vi "MultipleResultsPanelModel-GFV.vi"(8 "error in (no error)":errorcluster, 10 "Data in":variant, 11 "Enum":T1=enum."Init") -> (0 "error out":errorcluster, 3 "Data out":variant)   [LabVIEW 2013]
doc: "Use this template to build a VI to use as a subVI."
uses:
  TypeDef/MultipleResultsDataModel.ctl
  TypeDef/MultipleResultsModelOutput.ctl
  TypeDef/MultipleFilesModelInput.ctl
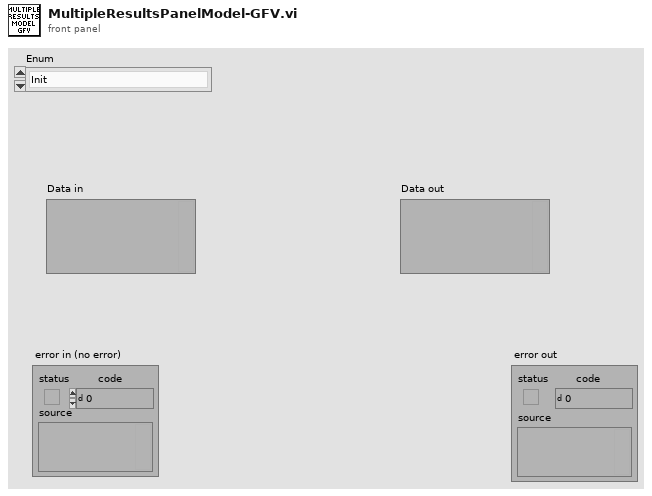
[diagram p1: front panel]
types:
  T1 = typedef "MultipleResultsDataModel.ctl" = enum16{"Get Results DB", "Get Plot Names", "Add Result File", "Init", "Get Input Data", "Get Result Graph Data", "Save Results DB", "Save Input Data"}
  T2 = typedef "MultipleResultsModelOutput.ctl" = cluster{"Ramp Pattern":dbl[], dbl[], "Include graph":bool, "Graph Name":string}[]
  T3 = typedef "MultipleFilesModelInput.ctl" = cluster{"Min Diameter (µm)":dbl, "Max Diameter (µm)":dbl, "FilterDropletsFrozeBelow":dbl, "Temperature offset for Calibration":dbl, "BinSizeDeg":dbl}
  T4 = cluster{"Values":dbl[][], "filename without extension":string}
  T5 = cluster{"Ramp Pattern":dbl[], dbl[], "Include graph":bool, "Graph Name":string}
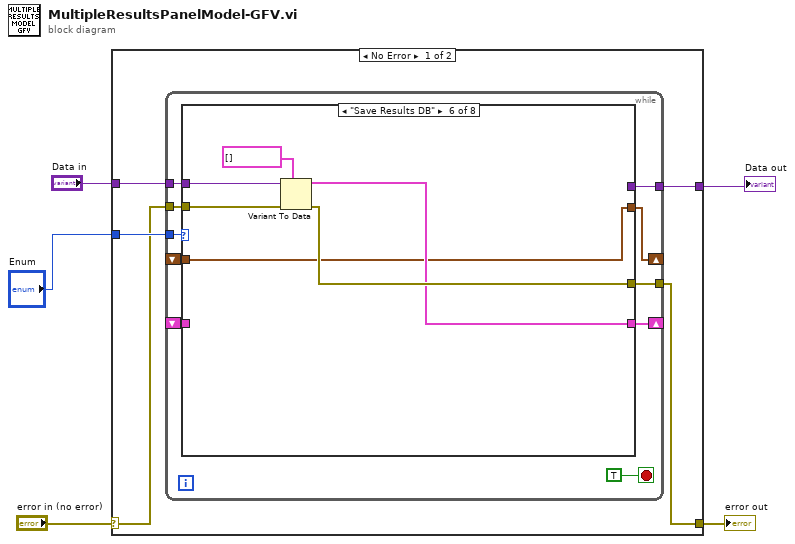
[diagram p0: block diagram]
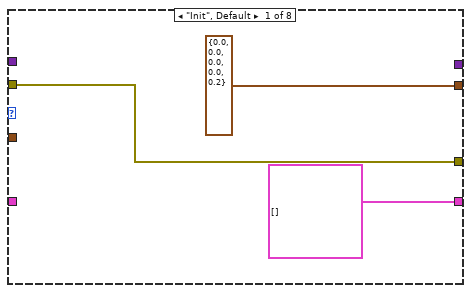
[diagram p2: hidden frame]
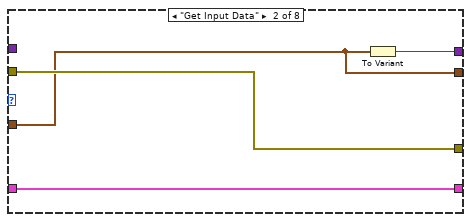
[diagram p3: hidden frame]
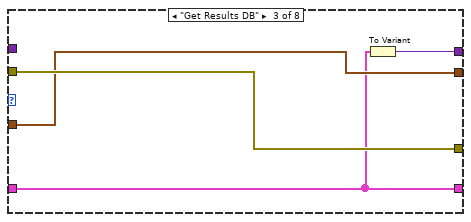
[diagram p4: hidden frame]
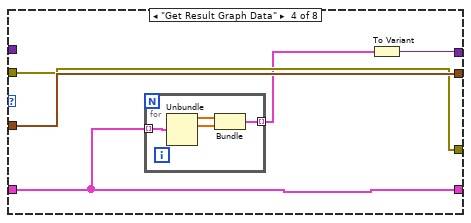
[diagram p5: hidden frame]
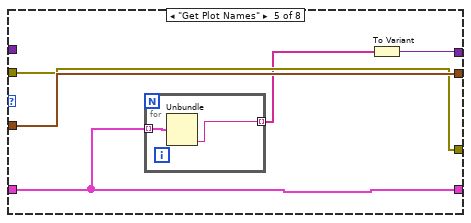
[diagram p6: hidden frame]
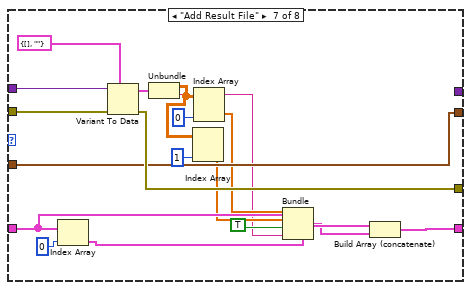
[diagram p7: hidden frame]
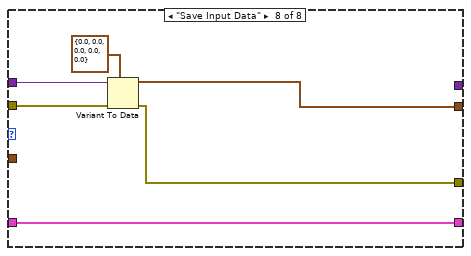
[diagram p8: hidden frame]
diagram:
  n1 = case shown="No Error" "error in (no error)" {
    selector: "error in (no error)" -> [w8 w78]
    tunnel: [w7 w78] -> w4
    tunnel: "Enum" -> [w10 _]
    tunnel: "Data in" -> [w9 _]
    tunnel: [w6 _] -> w2
    frame No Error {
      n2 = while {
        tunnel: w10 -> [w19]
        shift-right: [w18] -> _
        shift-left: _ -> [w14]
        tunnel: w9 -> [w17]
        tunnel: w8 -> [w16]
        tunnel: [w15] -> w7
        tunnel: [w13] -> w6
        shift-right: [w12] -> _
        shift-left: _ -> [w11]
        stop <- TRUE stop-if-true
        n3 = case shown="\"Save Results DB\"" w19 {
          tunnel: [T3 {"Min Diameter (µm)"=0.0, "Max Diameter (µm)"=0.0, "FilterDropletsFrozeBelow"=0.0, "Temperature offset for Calibration"=0.0, "BinSizeDeg"=0.2} w25 w29 w36 w45 w49 w68 w73] -> w18
          tunnel: w17 -> [_ _ _ _ _ w53 w71 w77]
          tunnel: w16 -> [w22 w26 w30 w35 w44 w52 w70 w76]
          tunnel: [w22 w26 w30 w35 w44 w51 w69 w75] -> w15
          tunnel: w14 -> [_ w25 w29 w36 w45 w49 w68 _]
          tunnel: [_ w27 w31 w34 w43 _ _ _] -> w13
          tunnel: [T2 [] ("Array") w24 w28 w33 w42 w50 w60 w72] -> w12
          tunnel: w11 -> [_ w24 w28 w33 w42 _ w62 w72]
          frame "Init", Default {
          }
          frame "Get Input Data" {
            n4 = To Variant(anything=w25) -> (Variant=w27:variant)
          }
          frame "Get Results DB" {
            n5 = To Variant(anything=w28) -> (Variant=w31:variant)
          }
          frame "Get Result Graph Data" {
            n6 = for {
              tunnel: w33 -> [w40] mode=indexing
              tunnel: [w37] -> w32 mode=indexing
              n7 = Unbundle(w40) -> ("Ramp Pattern"=w39:dbl[], w38:dbl[])  [unwired: 2 out]
              n8 = Bundle("Ramp Pattern"=w39, w38) -> (w37:cluster{"Ramp Pattern":dbl[], dbl[]})  [unwired: 1 in]
            }
            n9 = To Variant(anything=w32) -> (Variant=w34:variant)
          }
          frame "Get Plot Names" {
            n10 = for {
              tunnel: w42 -> [w47] mode=indexing
              tunnel: [w46] -> w41 mode=indexing
              n11 = Unbundle(w47) -> ("Graph Name"=w46:string)  [unwired: 3 out]
            }
            n12 = To Variant(anything=w41) -> (Variant=w43:variant)
          }
          frame "Save Results DB" {
            n13 = Variant To Data(error in=w52, type=T2 [] ("Normalized number of Droplets vs. Temperature"), Variant=w53) -> (data=w50:T2, error out=w51:errorcluster)
          }
          frame "Add Result File" {
            n14 = Index Array(array=w62, index=0) -> (element=w64:T5)
            n15 = Variant To Data(error in=w70, type=T4 {"Values"=[], "filename without extension"=""} ("output cluster"), Variant=w71) -> (data=w58:T4, error out=w69:errorcluster)
            n16 = Unbundle(w58) -> ("Values"=w57:dbl[][], "filename without extension"=w54:string)
            n17 = Index Array(array=w57, index (col)=1 ("disabled index (col)")) -> (element=w55:dbl[])  [unwired: 1 in]
            n18 = Index Array(array=w57, index (col)=0 ("disabled index (col)")) -> (element=w56:dbl[])  [unwired: 1 in]
            n19 = Bundle(cluster=w64, "Ramp Pattern"=w56, w55, "Include graph"=TRUE, "Graph Name"=w54) -> (w61:T5)
            n20 = Build Array (concatenate)(w62, w61) -> (w60:T2)
          }
          frame "Save Input Data" {
            n21 = Variant To Data(error in=w76, type=T3 {"Min Diameter (µm)"=0.0, "Max Diameter (µm)"=0.0, "FilterDropletsFrozeBelow"=0.0, "Temperature offset for Calibration"=0.0, "BinSizeDeg"=0.0}, Variant=w77) -> (data=w73:T3, error out=w75:errorcluster)
          }
        }
      }
    }
    frame Error {
    }
  }
  "error out" <- w4
  "Data out" <- w2
